vi "Write Lock-in configuration.vi"(8 "error in (no error)":errorcluster, 10 "Configuration":T1={"Frequency"=0.0, "Time constant"=0.0, "Synchronous"=FALSE, "Channels"=[1]} {"Time constant" format="%#_6ps"; "Frequency" format="%#_6pHz"}, 11 "Lock-in Driver in":refnum<class "Lock-in Driver.lvclass">) -> (0 "error out":errorcluster, 3 "Lock-in Driver out":refnum<class "Lock-in Driver.lvclass">)   [LabVIEW 2016, in "Lock-in Driver.lvclass"]
uses:
  Lock-in Driver.lvclass
  C:/github/NHMFL_Core/Libraries/Instruments/Instrument Driver/Instrument Driver.lvclass
  Lock-in Configuration.ctl
  Write User configuration.vi
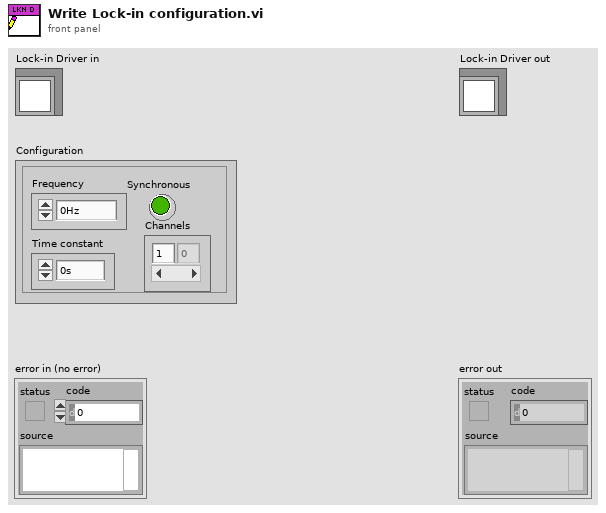
[diagram p1: front panel]
types:
  T1 = typedef "Lock-in Configuration.ctl" = cluster{"Frequency":dbl, "Time constant":dbl, "Synchronous":bool, "Channels":i32[]}
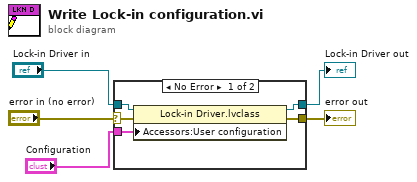
[diagram p0: block diagram]
diagram:
  n1 = case shown="No Error" "error in (no error)" {
    selector: "error in (no error)" -> [w10 w11]
    tunnel: [w9 w11] -> w4
    tunnel: [w7 w12] -> w2
    tunnel: "Lock-in Driver in" -> [w8 w12]
    tunnel: "Configuration" -> [w6 _]
    frame No Error {
      n2 = property class="Lock-in Driver.lvclass"(reference=w8, error in=w10, "Accessors:User configuration"=w6) -> (reference out=w7:refnum<class "Lock-in Driver.lvclass">, error out=w9:errorcluster)
    }
    frame Error {
    }
  }
  "error out" <- w4
  "Lock-in Driver out" <- w2
